vi "Set Address.vi"(6 "chip select (1st chip)":enum16{"1st chip", "2nd chip"}(ring), 8 "error in (no error)":errorcluster, 9 "address":u8 format="%.0x", 10 "address type (DDRAM)":enum16{"DDRAM", "CGRAM"}(ring), 11 "LCD in":u32) -> (0 "error out":errorcluster, 3 "LCD out":u32)   [LabVIEW 2015, in "HD44780 FPGA.lvlib"]
doc: "Sets the display data RAM (DDRAM) or character generator RAM (CGRAM) address."
uses:
  <vilib>/EmbeddedDisplay/Hitachi HD44780/FPGA/HD44780 FPGA.lvlib
  <vilib>/EmbeddedDisplay/Hitachi HD44780/Common/HD44780 Common.lvlib
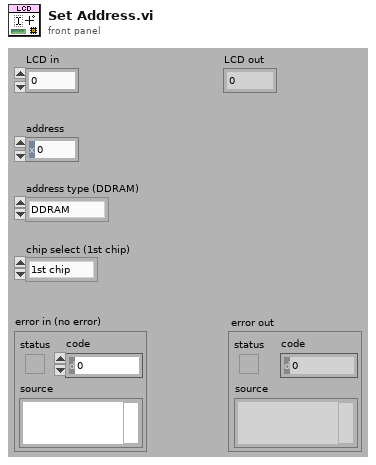
[diagram p1: front panel]
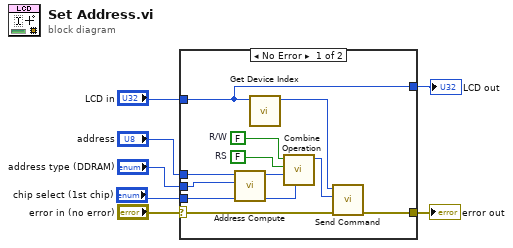
[diagram p0: block diagram]
diagram:
  n1 = case shown="No Error" "error in (no error)" {
    selector: "error in (no error)" -> [w14 w20]
    tunnel: [w10 w20] -> w6
    tunnel: "address" -> [w13 _]
    tunnel: "address type (DDRAM)" -> [w12 _]
    tunnel: "chip select (1st chip)" -> [w11 _]
    tunnel: "LCD in" -> [w8 w19]
    tunnel: [w8 w19] -> w1
    frame No Error {
      w17 = FALSE  # R/W
      w16 = FALSE  # RS
      n2 = call <vilib>:"Address Compute.vi"("address type (DD RAM)"=w12, "input address"=w13) -> ("output address"=w18:u8)  [unwired: 9 in]
      n3 = call <vilib>:"Get Device Index.vi"("LCD in"=w8) -> ("device index"=w9:i8)  [unwired: 10 in]
      n4 = call <vilib>:"Combine Operation.vi"("chip select  (1st chip)"=w11, "cmd/data (0)"=w18, "RS"=w16, "R/W"=w17) -> ("output"=w15:u32)  [unwired: 7 in]
      n5 = call <vilib>:"Send Command.vi"("error in (no error)"=w14, "operation"=w15, "device index"=w9) -> ("error out"=w10:errorcluster)  [unwired: 6 in, 2 out]
    }
    frame Error {
    }
  }
  "error out" <- w6
  "LCD out" <- w1
